vi "Thermal Chamber Controller_DQMH_Action Update Heater State-with-queue-teardown.vi"(8 "error in (no error)":errorcluster, 11 "test case ID":string) -> (3 "result":bool)   [LabVIEW 2018]
doc: "The teardown VI should be executed after the VI under test in the harness VI. In this VI you can evaluate the outputs of the VI under test.\n\nSee the Help Document for more information. (<b>Help</b> > <b>IncQuery Labs</b> > <b>InstaCoverage</b> > <b>InstaCoverage Help...</b>)"
uses:
  Libraries/Thermal Chamber Response Simulator/Thermal Chamber Response Simulator.lvlib
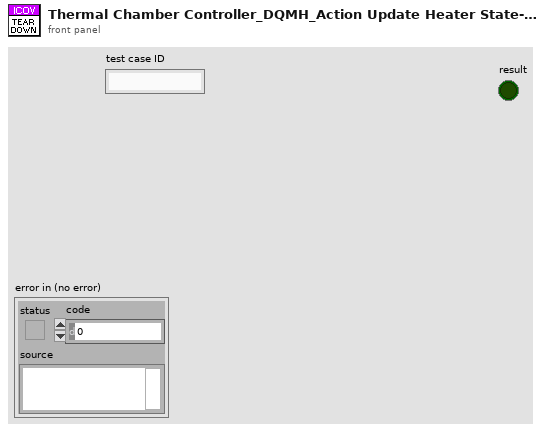
[diagram p1: front panel]
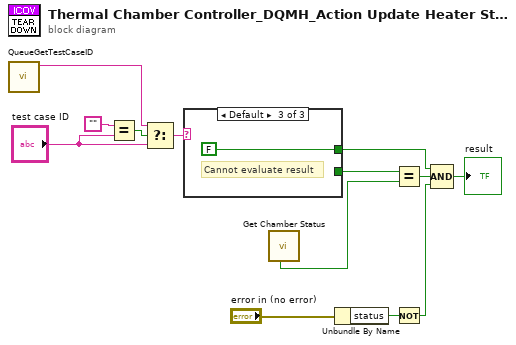
[diagram p0: block diagram]
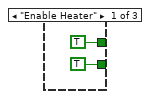
[diagram p2: hidden frame]
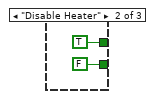
[diagram p3: hidden frame]
diagram:
  n1 = call "QueueGetTestCaseID.vi"() -> ("test case ID"=w5:string)  [unwired: 11 in]
  n2 = Equal?(x="", y="test case ID") -> (x = y?=w4:bool)
  n3 = Select(t=w5, s=w4, f="test case ID") -> (s? t:f=w1:string)
  n4 = case shown="Default" w1 {
    tunnel: [TRUE ("Heater State") FALSE ("Heater State") _] -> w11
    tunnel: [TRUE ("value") TRUE ("value") FALSE ("value")] -> w9
    frame "Enable Heater" {
    }
    frame "Disable Heater" {
    }
    frame Default {
      # "Cannot evaluate result"
    }
  }
  n5 = call "Get Chamber Status.vi"() -> ("Heater State"=w10:bool)  [unwired: 6 in, 5 out]
  n6 = Unbundle By Name("error in (no error)") -> ("status"=w7:bool)
  n7 = Equal?(x=w11, y=w10) -> (x = y?=w13:bool)
  n8 = Not(x=w7) -> (.not. x?=w6:bool)
  n9 = Compound Arithmetic op=AND(w9, w13, w6) -> (→"result":bool)
